vi "ProcImageHD_I8.vi"(5 "Digitizer Settings":T4={"Digitizer delay (us) "=0.0, "rf points per line"=2048, "lines per plane"=128, "Samp Rate (Hz)"=100000000.0, "Additional dig delay (us)"=0.0, "Voltage Scale"=0.4, "Pre-Looks"=0, "Offset delay (us)"=0.0, "bits A/D"=8, "Avg Num"=1, "DigTimeOut"=5.0, "Rel Dig Delay"=0.0, "Dig Ch"=0, "LeCroyCluster"={"LeCroy Channels"=[TRUE, FALSE, FALSE, FALSE], "LC read pt offset"=0.0, "Sweep Avg"=FALSE}, "Main Digitizer"=enum."NI Digitizer", "Dig Config"=enum."Single channel", "Digitizer ID Cluster"={"Acqiris/Alazar/SP ID"=[], "NI Instr Handles"=[], "LeCroy VISA"="", "GaGe Handle"={"Handle"=0, "Sample size"=0, "Resolution"=0, "Offset"=0, "Channels"=0, "Boards"=0}, "ATS Ref"="ATS9350", "Acqiris Address"=["PCI::INSTR0"], "ADQRef"=refnum, "adq_cu_ptr"=refnum}, "Trigger Settings"={"Trig Source"=1, "Trig Coupling"=0, "Trig Slope"=0, "Level (mV)"=1500.0}, "Bulk Acq"=FALSE, "Bulk Start Indexes"=[], "Data Ref RF"=refnum, "NI ID/Channel"=[], "Total Dig CH"=1, "Xtra Ann Trig delay (us)"=10.0, "Fix Z Delay?"=FALSE, "One Way Transmission?"=FALSE, "Data Ref Log"=refnum} {"Trigger Settings"."Trig Slope" items=["Positive", "Negative"]; "Trigger Settings"."Level (mV)" format="%.2f"; "Trigger Settings"."Trig Coupling" items=["DC 1 MOhm", "AC 1 MOhm", "DC 50 Ohm", "AC 50 Ohm"]; "Trigger Settings"."Trig Source" items=["Chan 1", "External"]; "Rel Dig Delay" format="%.2f"; "DigTimeOut" format="%.2f"; "Avg Num" min=1; "Offset delay (us)" format="%.2f"; "Additional dig delay (us)" format="%.2f"; "Digitizer delay (us)" format="%.2f"}, 6 "Ann Array Params":T1={"Synth Foc?"=FALSE, "Focal Zones"=41, "Switch T/R"=0, "Trans Geometry (mm)"={"Transducer"=0, "Geo Focus"=12.0, "a (radius)"=3.0, "# of rings"=5, "kerf space "=0.1, "Center Freq"=12.0}, "Sub Ap Excite?"=FALSE, "Full Array Scan?"=FALSE, "Xmt/Rcv"={"XMIT"=[TRUE, TRUE, TRUE, TRUE, TRUE], "RCV"=[TRUE, TRUE, TRUE, TRUE, TRUE]}, "PulseSpacing (us)"=0.0, "Xmit Ring"=0, "XMIT CHS"=0, "RCV CHS"=0, "GPU?"=FALSE, "Save TIFF?"=FALSE, "downfactor"=1, "RCV 1CH"=0} {"RCV 1CH" items=["All", "1", "2", "3", "4", "5"]; "Trans Geometry (mm)"."Transducer" items=["6D 12R 40 MHz"=0, "10D 31R 20 MHz"=1, "10D 23R 20 MHz"=2, "6D 23R 40 MHz"=3, "4.5D 10.7R 40 MHz"=4, "9D 23.5R 20 MHz"=5, "9D 25.8R 20MHz"=6, "Enter"=99]; "Switch T/R" min=1 max=5 step=1}, 7 "T/R Ring":i32, 8 "Scan Data In":i8[][](array[numeric]), 9 "Att (dB)":dbl) -> (0 "Synth App Out":i16[][](array[numeric]), 4 "Focal lengths":sgl[](array[numeric])=[0.0085, 0.009, 0.0095, 0.01, 0.0105, 0.011, 0.0115, 0.012, 0.0125, 0.013, 0.0135, 0.014, 0.0145, 0.015])   [LabVIEW 2022 SP3]
uses:
  ScanningControl/Digitizers/-DigitizerRoutines/DigitizerSettings.ctl
  ScanningControl/Digitizers/-DigitizerRoutines/Digitizer.ctl
  ScanningControl/Digitizers/-DigitizerRoutines/DigConfig.ctl
  ScanningControl/Digitizers/-DigitizerRoutines/DigitizerID.ctl
  C:/Windows/System32/ADQAPI_dotNet_helper.dll
  -AnnularRoutines/AnnularArray.ctl
  -AnnularRoutines/TransGeometry.ctl
  -AnnularRoutines/ArrayGeometry.ctl
  <vilib>/Analysis/baseanly.llb/Mean (DBL).vi
  ScanningControl/Motion Controllers/-MotionRoutines/MotionGlobals.vi
  <vilib>/Analysis/NI_AALBase.lvlib
panel:
  in  "One Way Receive":bool
  in  "Type of Mean":u16(ring) items=["Mean from lines", "Mean just lines", "Poly Mean", "No mean"]
  in  "Round to ROC?":bool
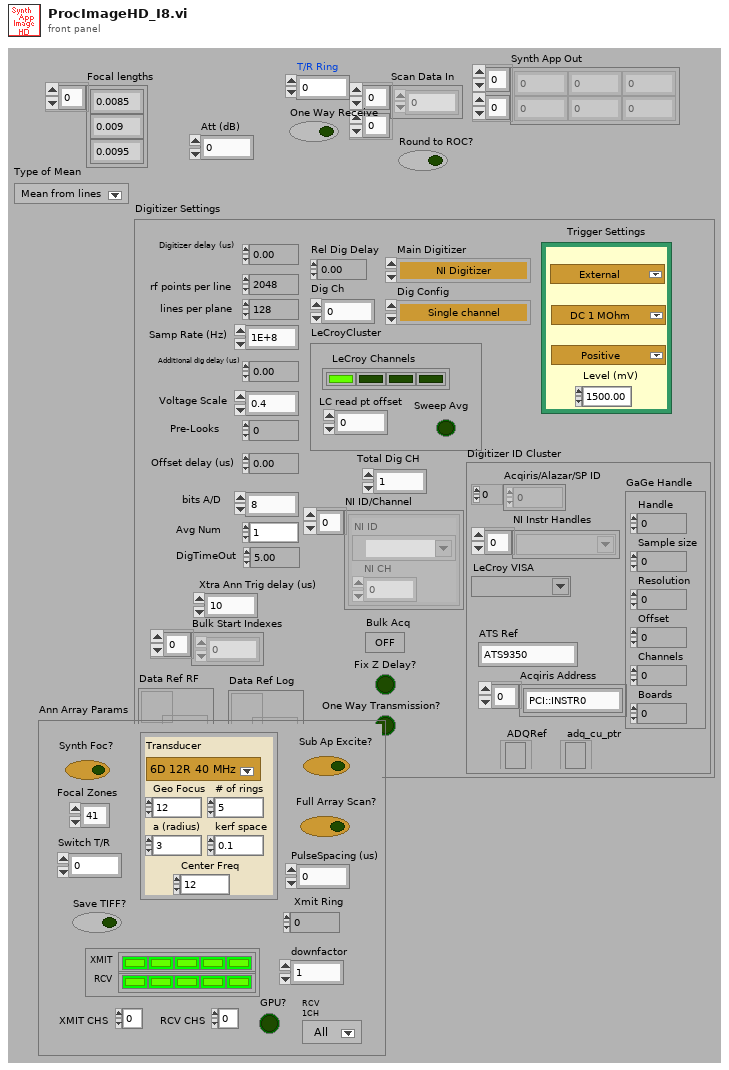
[diagram p1: front panel]
types:
  T1 = typedef "AnnularArray.ctl" = cluster{"Synth Foc?":bool, "Focal Zones":i16, "Switch T/R":i16, "Trans Geometry (mm)":T2, "Sub Ap Excite?":bool, "Full Array Scan?":bool, "Xmt/Rcv":cluster{"XMIT":bool[], "RCV":bool[]}, "PulseSpacing (us)":sgl, "Xmit Ring":i32, "XMIT CHS":u8, "RCV CHS":u8, "GPU?":bool, "Save TIFF?":bool, "downfactor":i32, "RCV 1CH":u16}
  T2 = typedef "TransGeometry.ctl" = cluster{"Transducer":T3, "Geo Focus":dbl, "a (radius)":dbl, "# of rings":i32, "kerf space ":dbl, "Center Freq":dbl}
  T3 = typedef "ArrayGeometry.ctl" = u16
  T4 = typedef "DigitizerSettings.ctl" = cluster{"Digitizer delay (us) ":dbl, "rf points per line":i32, "lines per plane":i32, "Samp Rate (Hz)":dbl, "Additional dig delay (us)":dbl, "Voltage Scale":dbl, "Pre-Looks":i32, "Offset delay (us)":dbl, "bits A/D":i8, "Avg Num":i32, "DigTimeOut":sgl, "Rel Dig Delay":sgl, "Dig Ch":i32, "LeCroyCluster":cluster{"LeCroy Channels":bool[], "LC read pt offset":dbl, "Sweep Avg":bool}, "Main Digitizer":T5, "Dig Config":T6, "Digitizer ID Cluster":T7, "Trigger Settings":cluster{"Trig Source":u16, "Trig Coupling":u16, "Trig Slope":u16, "Level (mV)":dbl}, "Bulk Acq":bool, "Bulk Start Indexes":i32[], "Data Ref RF":refnum<data-value>, "NI ID/Channel":cluster{"NI ID":refnum<k15>, "NI CH":i32}[], "Total Dig CH":i32, "Xtra Ann Trig delay (us)":dbl, "Fix Z Delay?":bool, "One Way Transmission?":bool, "Data Ref Log":refnum<data-value>}
  T5 = typedef "Digitizer.ctl" = enum16{"Acqiris Digitizer", "NI Digitizer", "LeCroy", "GaGe", "AlazarTech", "No Digitizer", "Teledyne"}
  T6 = typedef "DigConfig.ctl" = enum16{"Single channel", "2 Chans w/ 2 Acqiris", "2 Chans w/ 1 Acqiris", "5-CH Pulser New", "5-CH pulser w/ ann array", "5-pass style ann array", "Empty"}
  T7 = typedef "DigitizerID.ctl" = cluster{"Acqiris/Alazar/SP ID":u32[], "NI Instr Handles":refnum<k15>[], "LeCroy VISA":refnum<visa-resource-name>, "GaGe Handle":cluster{"Handle":u32, "Sample size":u32, "Resolution":i32, "Offset":i32, "Channels":u32, "Boards":u32}, "ATS Ref":string, "Acqiris Address":string[], "ADQRef":refnum<k24>, "adq_cu_ptr":refnum<k24>}
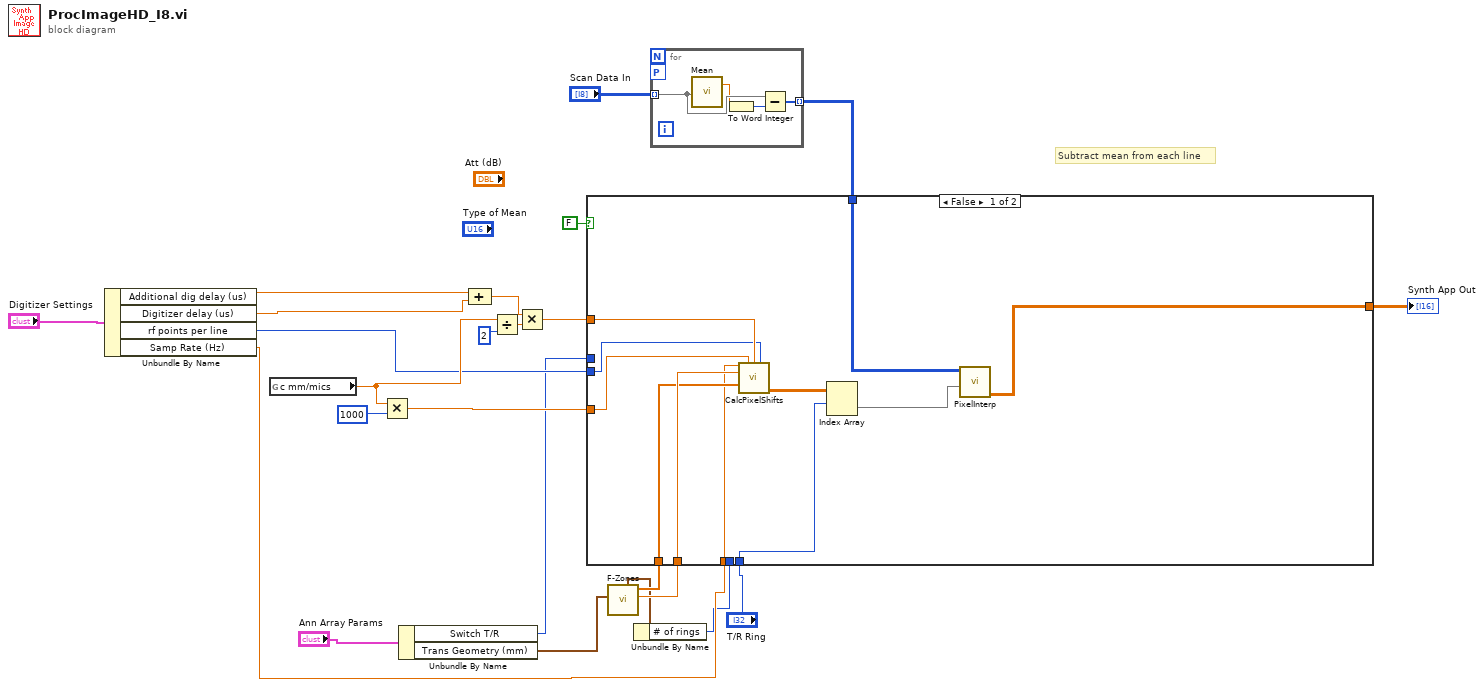
[diagram p0: block diagram]
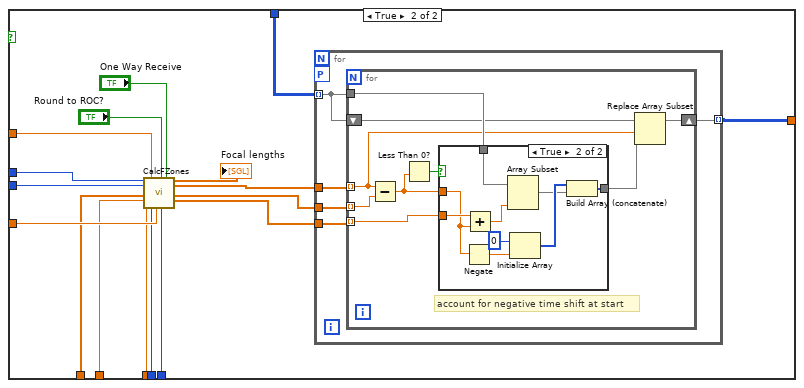
[diagram p2: hidden frame]
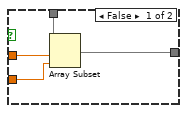
[diagram p3: hidden frame]
diagram:
  # "Subtract mean from each line"
  n1 = Unbundle By Name("Digitizer Settings") -> ("Additional dig delay (us)"=w11:dbl, "Digitizer delay (us)"=w10:dbl, "rf points per line"=w9:i32, "Samp Rate (Hz)"=w8:dbl)
  n2 = global read "MotionGlobals.vi" "c mm/mics"() -> (w14:sgl)
  n3 = Multiply(x=w14, y=1000) -> (x*y=w21:sgl)
  n4 = Unbundle By Name("Ann Array Params") -> ("Switch T/R"=w2:i16, "Trans Geometry (mm)"=w3:T2)
  n5 = Compound Arithmetic op=ADD(w11, w10) -> (w12:dbl)
  n6 = Divide(x=w14, y=2) -> (x/y=w23:sgl)
  n7 = Multiply(x=w12, y=w23) -> (x*y=w13:dbl)
  n8 = call "F-Zones.vi"("Trans Geometry (mm)"=w3) -> ("ROC (m)"=w19:dbl, "annuli rad (m)"=w20:dbl[], "Trans Geometry (mm) out"=w6:T2)  [unwired: 7 in, 1 out]
  n9 = Unbundle By Name(w6) -> ("# of rings"=w5:i32)
  n10 = for {
    tunnel: "Scan Data In" -> [w28] mode=indexing
    tunnel: [w27] -> w15 mode=indexing
    workers-P: _ -> [_]
    n11 = call-poly <vilib>:"Mean.vi"("X"=w28) -> ("mean"=w26:dbl)  [unwired: 1 out]
    n12 = To Word Integer(number=w26) -> (16bit integer=w25:i16)
    n13 = Subtract(x=w28, y=w25) -> (x-y=w27:i16[])
  }
  n14 = case shown="False" FALSE {
    tunnel: w21 -> [w33 w55]
    tunnel: w20 -> [w35 w53]
    tunnel: w19 -> [w36 w52]
    tunnel: "T/R Ring" -> [w30 w51]
    tunnel: [w31 w49] -> w17
    tunnel: w15 -> [w32 w48]
    tunnel: w13 -> [w37 w47]
    tunnel: w9 -> [w34 w43]
    tunnel: w8 -> [w29 w42]
    tunnel: w5 -> [_ w41]
    tunnel: w2 -> [_ w40]
    frame False {
      n15 = call "CalcPixelShifts.vi"("Sampling Rate (Hz)"=w29, "c (m/s)"=w33, "delay (mm)"=w37, "rf pts"=w34, "ROC (m)"=w36, "Radii (m)"=w35) -> ("InterpIndex"=w39:sgl[][])  [unwired: 9 in]
      n16 = Index Array(array=w39, index (row)=w30) -> (element=w38:sgl[])  [unwired: 1 in]
      n17 = call "PixelInterp.vi"("IndexVals"=w38, "Array data"=w32) -> ("Synth App Out"=w31:dbl[][])  [unwired: 6 in]
    }
    frame True {
      n18 = call "CalcFZones.vi"("F- zones"=w40, "# rf points per line"=w43, "Radii (m)"=w53, "ROC (m)"=w52, "Sampling Rate"=w42, "delay (mm)"=w47, "# Elements"=w41, "c (m/s)"=w55, "Round to ROC?"="Round to ROC?", "File index number"=w51, "One Way Receive"="One Way Receive") -> ("FZones (m)"=→"Focal lengths":dbl[], "ZoneStart"=w44:sgl[], "ZoneShift"=w45:sgl[], "ZoneLength"=w46:sgl[])  [unwired: 3 in, 2 out]
      n19 = for {
        tunnel: w48 -> [w61] mode=indexing
        tunnel: w44 -> [w60]
        tunnel: w45 -> [w59]
        tunnel: w46 -> [w58]
        workers-P: _ -> [_]
        tunnel: [w57] -> w49 mode=indexing
        n20 = for {
          tunnel: w60 -> [w63] mode=indexing
          tunnel: w58 -> [w70] mode=indexing
          tunnel: w59 -> [w69] mode=indexing
          tunnel: w61 -> [w66]
          shift-right: [w65] -> w57
          shift-left: w61 -> [w64]
          # "account for negative time shift at start"
          n21 = Subtract(x=w63, y=w69) -> (x-y=w67:sgl)
          n22 = Less Than 0?(x=w67) -> (x < 0?=w68:bool)
          n23 = case shown="True" w68 {
            tunnel: w66 -> [w74 w82]
            tunnel: w70 -> [w72 w83]
            tunnel: [w73 w77] -> w62
            tunnel: w67 -> [w71 w80]
            frame False {
              n24 = Array Subset(array=w74, index=w71, length=w72) -> (w73:i16[])
            }
            frame True {
              n25 = Negate(x=w80) -> (-x=w75:sgl)
              n26 = Add(x=w83, y=w80) -> (x+y=w76:sgl)
              n27 = Array Subset(array=w82, length=w76) -> (w78:i16[])  [unwired: 1 in]
              n28 = Initialize Array(i16 0, w75) -> (w79:i16[])
              n29 = Build Array (concatenate)(w79, w78) -> (w77:i16[])
            }
          }
          n30 = Replace Array Subset(array=w64, new element=w62, index=w63) -> (w65:i16[])
        }
      }
    }
  }
  "Synth App Out" <- w17
